vi "String_Covert Character to Serachable Character.vi"(4 "Char":string) -> (1 "Searchable Char Out":string)   [LabVIEW 2015]
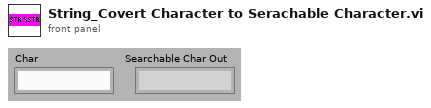
[diagram p1: front panel]
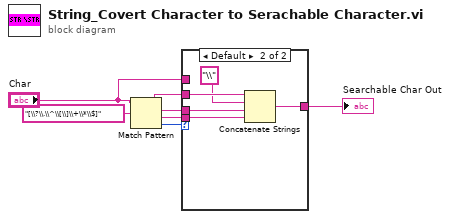
[diagram p0: block diagram]
diagram:
  n1 = Match Pattern(string="Char", regular expression="[\\?\\.\\^\\[\\]\\+\\*\\$]") -> (before substring=w6:string, match substring=w3:string, after substring=w5:string, offset past match=w2:i32)  [unwired: 1 in]
  n2 = case shown="Default" w2 {
    tunnel: w6 -> [_ w13]
    tunnel: w5 -> [_ w12]
    tunnel: [w8 w11] -> w4
    tunnel: w3 -> [_ w9]
    tunnel: "Char" -> [w8 _]
    frame -1 {
    }
    frame Default {
      n3 = Concatenate Strings(w13, "\\", w9, w12) -> (w11:string)
    }
  }
  "Searchable Char Out" <- w4
